vi "Msg.vi"(7 "Actor in":refnum<class "Actor.lvclass">, 11 "Teardown Msg in":refnum<class "Teardown Msg.lvclass">) -> (5 "Actor out":refnum<class "Actor.lvclass">)   [LabVIEW 2020, in "jettl.lvlib" / "Teardown Msg.lvlib" / "Teardown Msg.lvclass"]
uses:
  Teardown Msg.lvclass
  Actor/Actor/Actor.lvclass
  Teardown/Teardown.lvclass
  Teardown Msg.lvclass/Teardown Msg.ctl
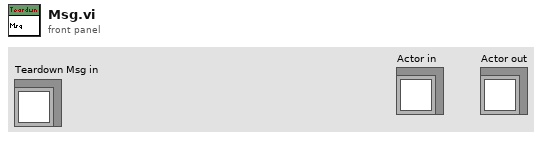
[diagram p1: front panel]
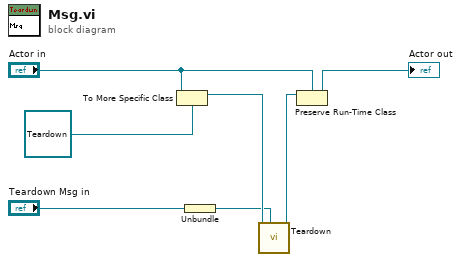
[diagram p0: block diagram]
diagram:
  n1 = To More Specific Class(target class=refnum<class "Teardown.lvclass"> refnum ("Destroy.lvlib:Destroy.lvclass"), reference="Actor in") -> (specific class reference=w3:refnum<class "Teardown.lvclass">)  [unwired: 1 in, 1 out]
  n2 = Unbundle "Unbundle"("Teardown Msg in") -> (w1:refnum<class "Sender.lvclass">)
  n3 = call-dynamic "Teardown.vi"("Sender"=w1, "Teardown in"=w3) -> ("Teardown out"=w2:refnum<class "Teardown.lvclass">)  [unwired: 9 in]
  n4 = Preserve Run-Time Class(object in=w2, 2:"Actor in") -> (object out=→"Actor out":refnum<class "Actor.lvclass">)  [unwired: 1 in, 1 out]
